vi "Launcher_Template.vi"   [LabVIEW 2020]
uses:
  Actor_Controller_Template/Actor_Controller_Template/Actor_Controller_Template.lvclass
  C:/Program Files/National Instruments/LabVIEW 2020/vi.lib/ActorFramework/Actor/Actor.lvclass
  <vilib>/ActorFramework/Actor/Actor.lvclass
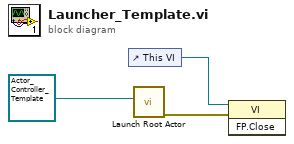
[diagram p0: block diagram]
diagram:
  n1 = control-ref of="This VI"() -> (w1:refnum<vi>)
  n2 = call <vilib>:"Launch Root Actor.vi"("Actor"=refnum<class "Actor_Controller_Template.lvclass"> refnum ("Actor_Controller_Template.lvlib:Actor_Controller_Template.lvclass")) -> ("error out"=w2:errorcluster)  [unwired: 9 in, 1 out]
  n3 = invoke class="VI" method="FP.Close"(reference=w1, error in=w2) -> ()  [unwired: 1 in, 3 out]
